vi "TMP007 Init.vi"(7 "I2C Channel":u8, 8 "error in (no error)":errorcluster, 9 "Samples to Average":u16(ring) items=["1 sample, .26s conversion"=0, "2 samples, .51s conversion"=512, "4 samples, 1.01s conversion"=1024, "8 samples, 2.01s conversion"=1536, "16 samples, 4.01s conversion"=2048], 10 "I2C Slave Address":u8=64 format="%.0x", 11 "LINX Resource in":T3) -> (0 "error out":errorcluster, 1 "Thermopile Setting":T1 {"Last Temp Readings"."Ambient Temp (°F)" format="%.2f °F"; "Last Temp Readings"."Ambient Temp (°C)" format="%.2f °C"; "Last Temp Readings"."Object Temp (°F)" format="%.2f °F"; "Last Temp Readings"."Object Temp (°C)" format="%.2f °C"; "Samples to Average" items=["1 sample, .26s conversion"=0, "2 samples, .51s conversion"=512, "4 samples, 1.01s conversion"=1024, "8 samples, 2.01s conversion"=1536, "16 samples, 4.01s conversion"=2048]; "I2C Slave Address" format="%.0x"}, 3 "LINX Resource out":T3)   [LabVIEW 2018]
uses:
  <vilib>/MakerHub/LINX/Private/Type Defs/Platform.ctl
  <vilib>/MakerHub/LINX/Private/Type Defs/Interface.ctl
  <vilib>/MakerHub/LINX/Private/Device/Type Defs/TCP Config.ctl
  <vilib>/MakerHub/LINX/Private/Device/Type Defs/Channels.ctl
  <vilib>/MakerHub/LINX/Private/Device/Type Defs/LINX Device Config.ctl
  <vilib>/MakerHub/LINX/Private/Type Defs/LINX Ref.ctl
  Type Defs/thermopileSettings.ctl
  Type Defs/tempReadings.ctl
panel:
  # "Each sample takes .25s to convert\nThere are some other conversion modes that include idle times, but I didn't include those modes"
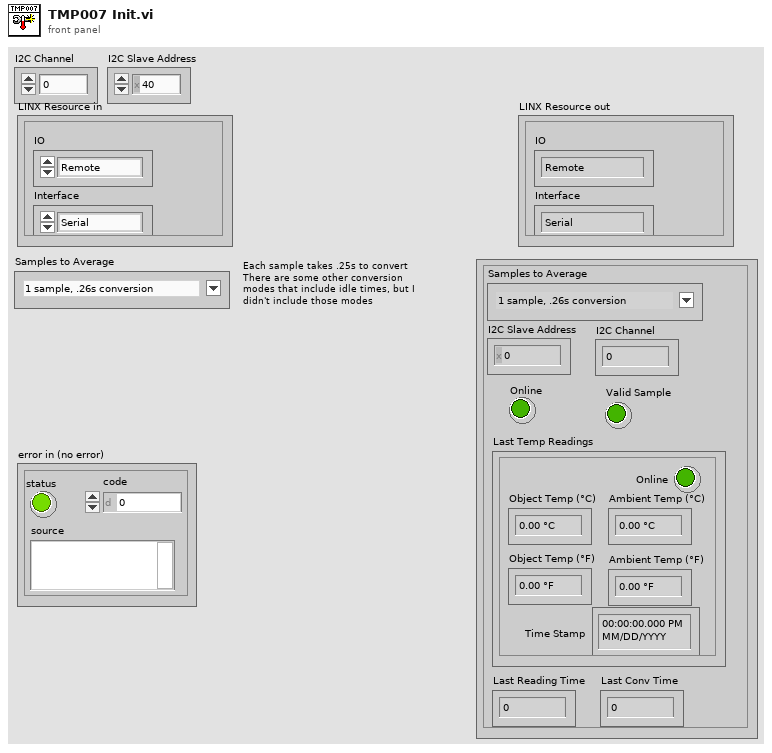
[diagram p1: front panel]
types:
  T1 = typedef "thermopileSettings.ctl" = cluster{"Online":bool, "I2C Channel":u8, "I2C Slave Address":u8, "Valid Sample":bool, "Samples to Average":u16, "Last Temp Readings":T2, "Last Reading Time":dbl, "Last Conv Time":dbl}
  T2 = typedef "tempReadings.ctl" = cluster{"Object Temp (°C)":dbl, "Object Temp (°F)":dbl, "Ambient Temp (°C)":dbl, "Ambient Temp (°F)":dbl, "Online":bool, "Time Stamp":timestamp}
  T3 = typedef "LMH-LINX.lvlib/LINX Ref.ctl" = cluster{"IO":T4, "Interface":T5, "LINX Device Config":T6}
  T4 = typedef "LMH-LINX.lvlib/Platform.ctl" = enum16{"Remote", "Local"}
  T5 = typedef "LMH-LINX.lvlib/Interface.ctl" = enum16{"Serial", "TCP"}
  T6 = typedef "LMH-LINX.lvlib/Device.lvlib/LINX Device Config.ctl" = cluster{"Interface":T5, "COM Port":refnum<visa-resource-name>, "TCP Configuration":T7, "Device Family":u8, "Device ID":u8, "Device Name":string, "TCP Ref":refnum<k5>, "Channels":T8}
  T7 = typedef "LMH-LINX.lvlib/Device.lvlib/TCP Config.ctl" = cluster{"IP Address":string, "Port":u16}
  T8 = typedef "LMH-LINX.lvlib/Channels.ctl" = cluster{"DI":u8[], "DO":u8[], "AI":u8[], "AO":u8[], "PWM":u8[], "QE":u8[], "UART":u8[], "I2C 2":u8[], "SPI":u8[], "CAN":u8[], "Servo":u8[], "AI Ref (V)":dbl, "AI Resolution (Bits)":u8, "AO Ref (V)":dbl, "AO Resolution (Bits)":u8}
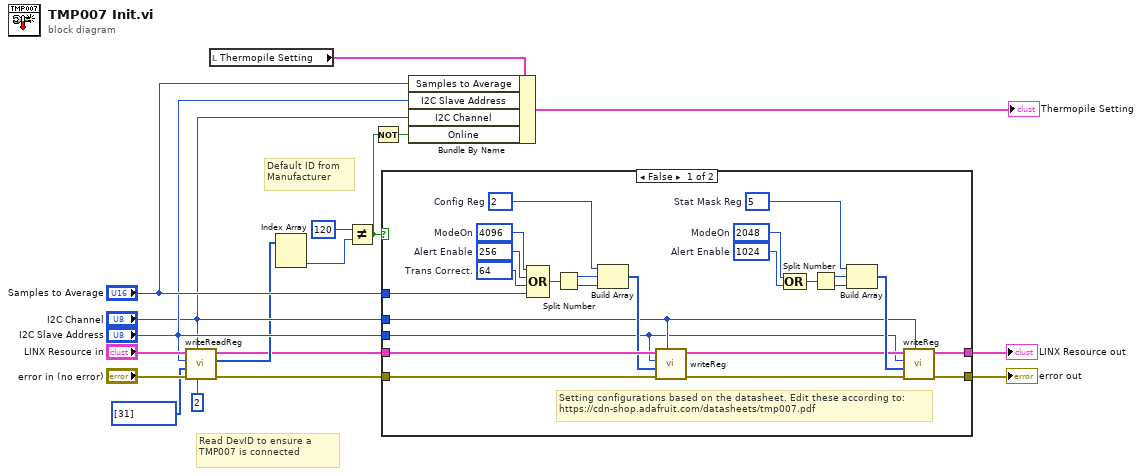
[diagram p0: block diagram]
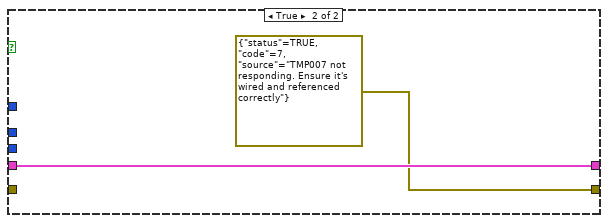
[diagram p2: hidden frame]
diagram:
  # "Default ID from Manufacturer"
  # "Read DevID to ensure a TMP007 is connected"
  n1 = call "writeReadReg.vi"("Bytes To Read"=u8 2, "I2C Channel"="I2C Channel", "error in"="error in (no error)", "Data"=u8[] [31], "I2C Slave Address"="I2C Slave Address", "LINX Resource in"="LINX Resource in") -> ("error out"=w2:errorcluster, "Bytes Read"=w4:u8[], "LINX Resource out"=w3:T3)  [unwired: 3 in]
  n2 = local read "Thermopile Setting"() -> (w11:T1)
  n3 = Index Array(array=w4) -> (element #2=w12:u8)  [unwired: 2 in, 1 out]
  n4 = Not Equal?(x=u8 120, y=w12) -> (x != y?=w7:bool)
  n5 = Not(x=w7) -> (.not. x?=w1:bool)
  n6 = case shown="False" w7 {
    tunnel: w3 -> [w42 w44]
    tunnel: [w20 w44] -> w17
    tunnel: w2 -> [w41 _]
    tunnel: [w19 errorcluster {"status"=TRUE, "code"=7, "source"="TMP007 not responding. Ensure it's wired and referenced correctly"} ("error constant")] -> w16
    tunnel: "Samples to Average" -> [w40 _]
    tunnel: "I2C Channel" -> [w22 _]
    tunnel: "I2C Slave Address" -> [w21 _]
    frame False {
      w31 = u8 5  # Stat Mask Reg
      w26 = u16 1024  # Alert Enable
      w27 = u16 2048  # ModeOn
      w33 = u8 2  # Config Reg
      w39 = u16 64  # Trans Correct.
      w38 = u16 256  # Alert Enable
      w37 = u16 4096  # ModeOn
      # "Setting configurations based on the datasheet. Edit these according to:\nhttps://cdn-shop.adafruit.com/datasheets/tmp007.pdf"
      n7 = Compound Arithmetic op=OR(w37, w38, w39, w40) -> (w36:u16)
      n8 = Split Number(x=w36) -> (hi(x)=w35:u8, lo(x)=w34:u8)
      n9 = Build Array(w33, w35, w34) -> (w32:u8[])
      n10 = call "writeReg.vi"("I2C Channel"=w22, "error in"=w41, "Data"=w32, "I2C Slave Address"=w21, "LINX Resource in"=w42) -> ("error out"=w23:errorcluster, "LINX Resource"=w24:T3)  [unwired: 5 in]
      n11 = Compound Arithmetic op=OR(w27, w26) -> (w28:u16)
      n12 = Split Number(x=w28) -> (hi(x)=w29:u8, lo(x)=w30:u8)
      n13 = Build Array(w31, w29, w30) -> (w25:u8[])
      n14 = call "writeReg.vi"("I2C Channel"=w22, "error in"=w23, "Data"=w25, "I2C Slave Address"=w21, "LINX Resource in"=w24) -> ("error out"=w19:errorcluster, "LINX Resource"=w20:T3)  [unwired: 5 in]
    }
    frame True {
    }
  }
  "error out" <- w16
  "LINX Resource out" <- w17
  n15 = Bundle By Name(cluster=w11, "Samples to Average"="Samples to Average", "I2C Slave Address"="I2C Slave Address", "I2C Channel"="I2C Channel", "Online"=w1) -> (→"Thermopile Setting":T1)
